vi "Misorientation to Interface Plane parameters.vi"(9 "Misorientation Angle":dbl=60.0, 10 "Misorientation Axis, o":dbl[](array[numeric])=[1.0, 1.0, 1.0], 11 "Grain 1 Orientation":dbl[](array[numeric])=[1.0, 1.0, 1.0]) -> (0 "Misorientation Matrix":T1, 1 "Tilt Angle (Deg)":dbl, 2 "Twist Angle (Deg)":dbl, 3 "Grain 2 Orientation":dbl[](array[numeric])=[1.0, 1.0, 1.0])   [LabVIEW 2010]
uses:
  <vilib>/Analysis/Matrix/Datatypes/RealMatrix.ctl
  <vilib>/Analysis/baseanly.llb/A x Vector.vi
  <vilib>/Analysis/NI_AALBase.lvlib
  <vilib>/Analysis/Matrix/NI_Matrix.lvlib
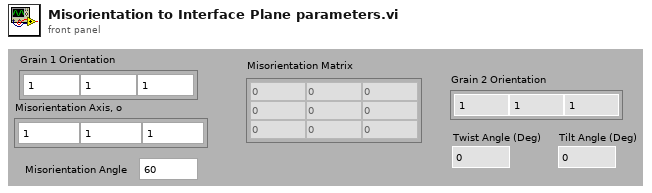
[diagram p1: front panel]
types:
  T1 = typedef "NI_Matrix.lvlib/RealMatrix.ctl" = dbl[][]
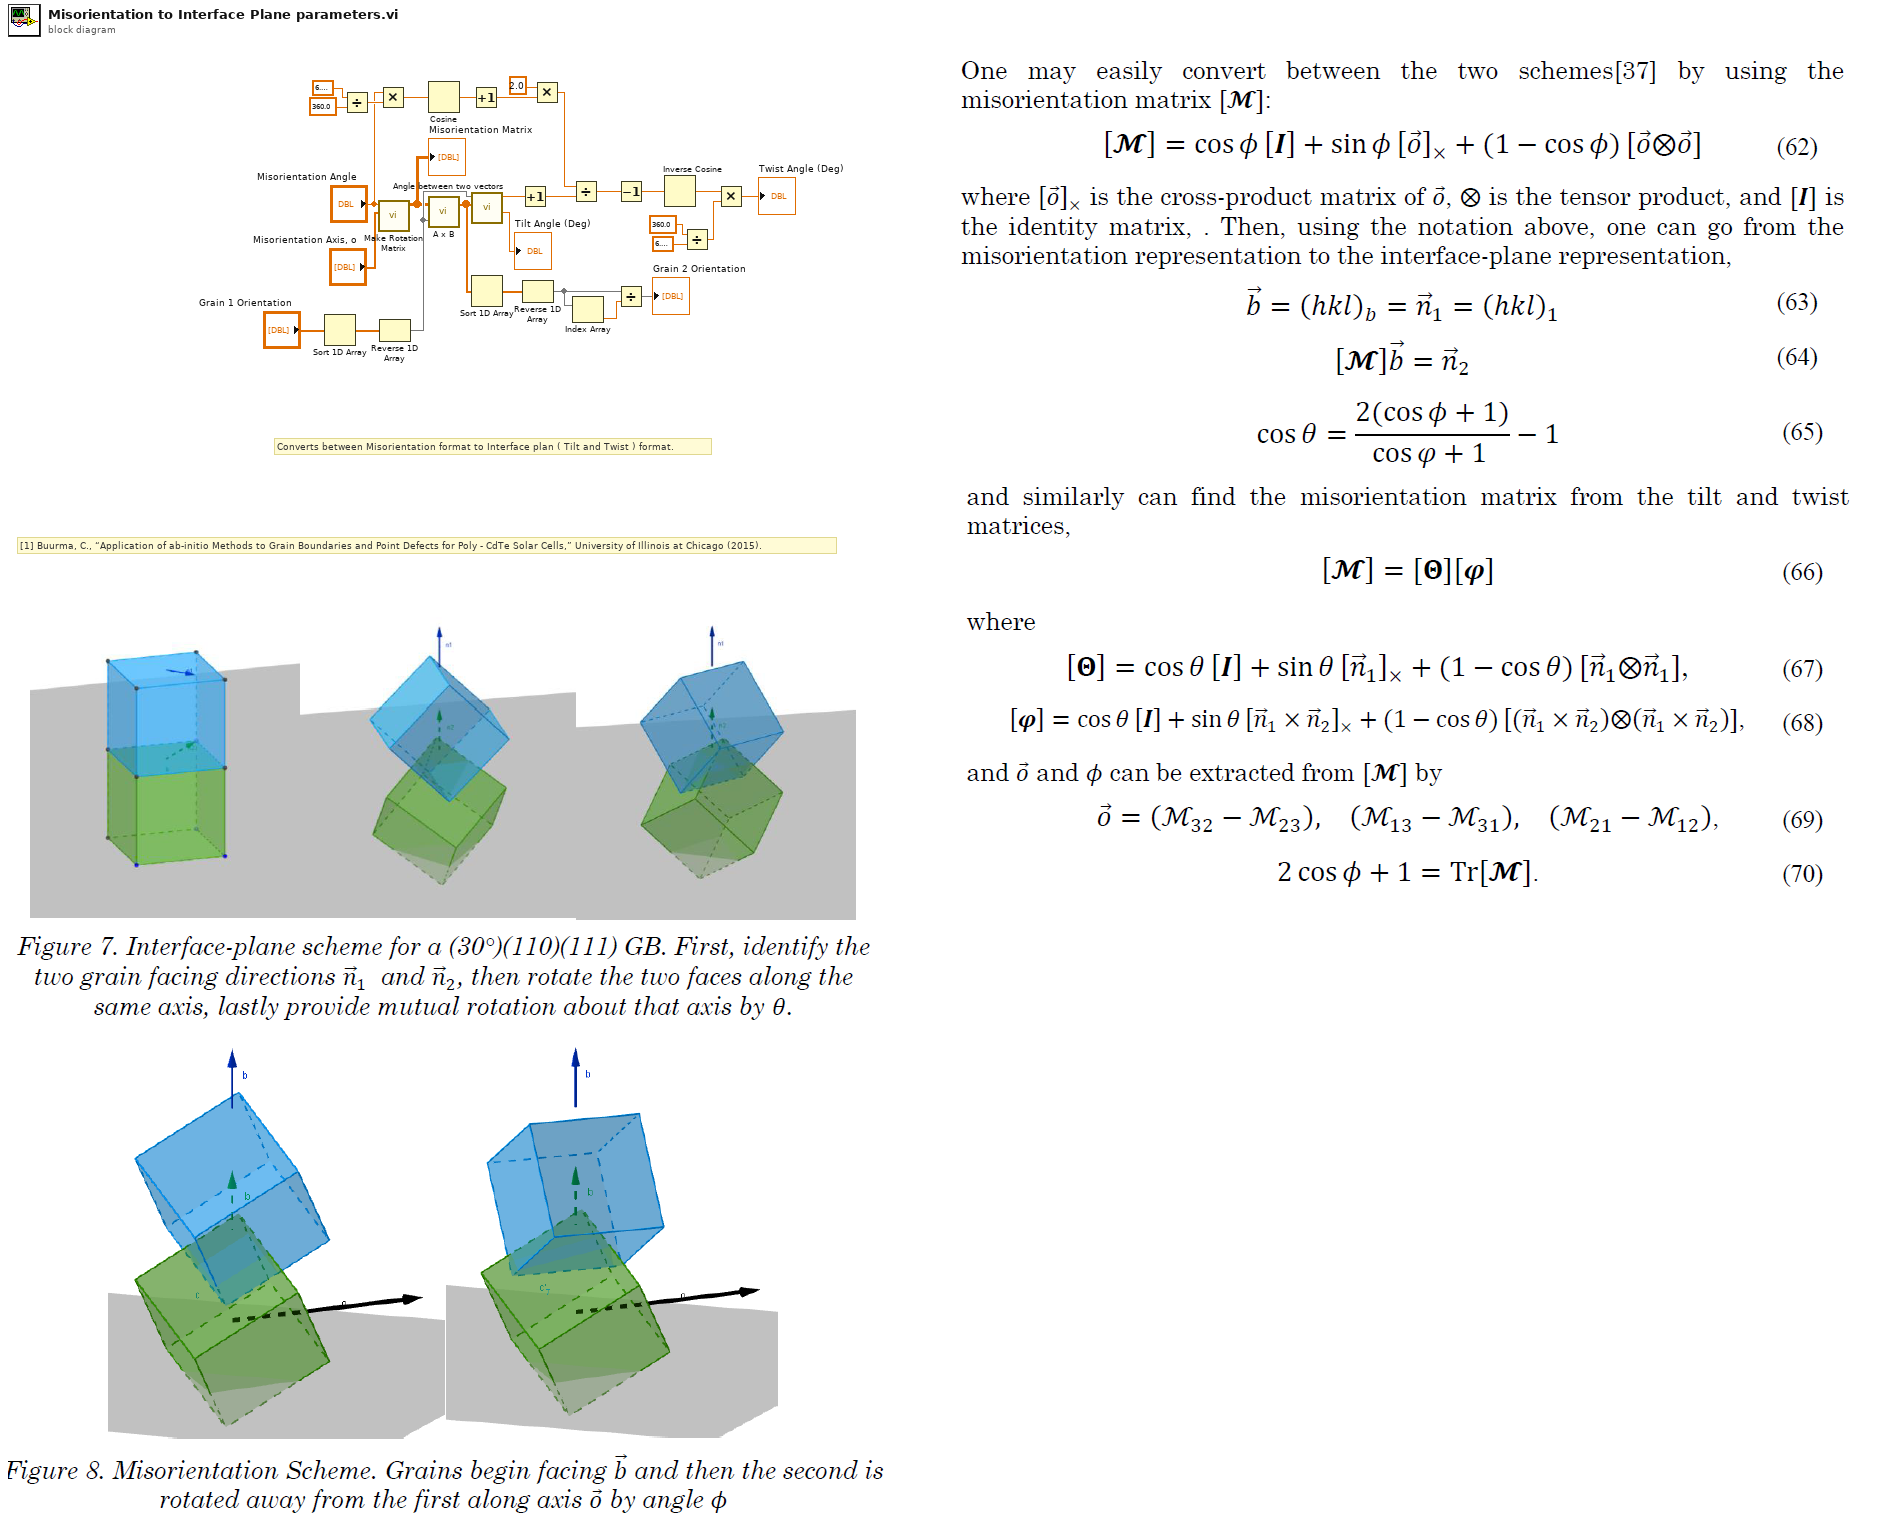
[diagram p0: block diagram]
diagram:
  # "[1] Buurma, C., “Application of ab-initio Methods to Grain Boundaries and Point Defects for Poly - CdTe Solar Cells,” University of Illinois at Chicago (2015)."
  # "Converts between Misorientation format to Interface plan ( Tilt and Twist ) format."
  n1 = Sort 1D Array(array="Grain 1 Orientation") -> (sorted array=w29:dbl[])
  n2 = Divide(x=6.283185307179586, y=360.0 ("x")) -> (x/y=w10:dbl)
  n3 = Multiply(x="Misorientation Angle", y=w10) -> (x*y=w6:dbl)
  n4 = call "Make Rotation Matrix.vi"("Rotation Axis"="Misorientation Axis, o", "Rotation Angle (Degree)"="Misorientation Angle") -> ("Rotation Matrix"=w25:T1)  [unwired: 9 in]
  "Misorientation Matrix" <- w25
  n5 = Reverse 1D Array(array=w29) -> (reversed array=w26:dbl[])
  n6 = Cosine(x=w6) -> (cos(x)=w23:dbl)
  n7 = call-poly <vilib>:"A x B.vi"("Vector"=w26, "A"=w25) -> ("A x Vector"=w5:dbl[])  [unwired: 1 out]
  n8 = Increment(x=w23) -> (x+1=w22:dbl)
  n9 = call "Angle between two vectors.vi"("Vector 2"=w5, "Vector 1"=w26) -> ("Angle (Degrees)"=→"Tilt Angle (Deg)":dbl, "Cos (Theta)"=w11:dbl)  [unwired: 7 in, 1 out]
  n10 = Sort 1D Array(array=w5) -> (sorted array=w4:dbl[])
  n11 = Increment(x=w11) -> (x+1=w20:dbl)
  n12 = Reverse 1D Array(array=w4) -> (reversed array=w3:dbl[])
  n13 = Multiply(x=2.0, y=w22) -> (x*y=w21:dbl)
  n14 = Divide(x=w21, y=w20) -> (x/y=w18:dbl)
  n15 = Index Array(array=w3) -> (element=w2:dbl)  [unwired: 1 in]
  n16 = Decrement(x=w18) -> (x-1=w12:dbl)
  n17 = Divide(x=w3, y=w2) -> (x/y=→"Grain 2 Orientation":dbl[])
  n18 = Inverse Cosine(1:w12) -> (0:w17:dbl)
  n19 = Divide(x=360.0, y=6.283185307179586) -> (x/y=w14:dbl)
  n20 = Multiply(x=w17, y=w14) -> (x*y=→"Twist Angle (Deg)":dbl)
